vi "Private AdsSymbolVersionChanged Event Callback.vi"(4 "TwinCAT ADS out":refnum<class "TwinCAT ADS.lvclass">, 5 "Event Data":cluster{"sender":refnum<k24>, "e":refnum<k24>}, 6 "Control Ref":refnum<k24>, 7 "Event Common Data":T1) -> ()   [LabVIEW 2018, in "TwinCAT ADS.lvclass"]
uses:
  TwinCAT ADS.lvclass
  TwinCAT.Ads
  TwinCAT ADS.lvclass/TwinCAT ADS.ctl
  <vilib>/event_ctls.llb/usereventprio.ctl
  Get Type Map.vi
  From Notification Key.vi
  Get Notification Map.vi
  Extensions/Delete Notification By Handle.vi
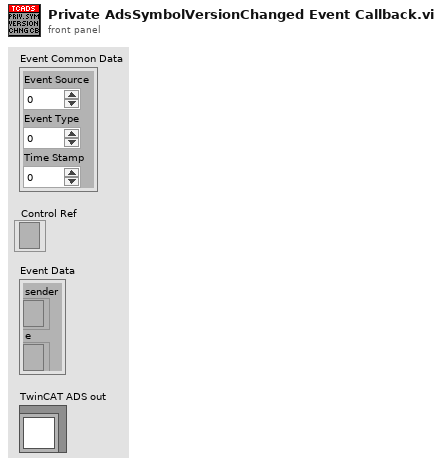
[diagram p1: front panel]
types:
  T1 = cluster{"Event Source":i32, "Event Type":u32, "Time Stamp":u32}
  T2 = typedef "usereventprio.ctl" = enum32{"high priority", "normal priority"}
  T3 = typedef "TwinCAT ADS.lvclass/Notifcation Map Value.ctl" = cluster{"Handle":i32, "Cycle Time":i32}
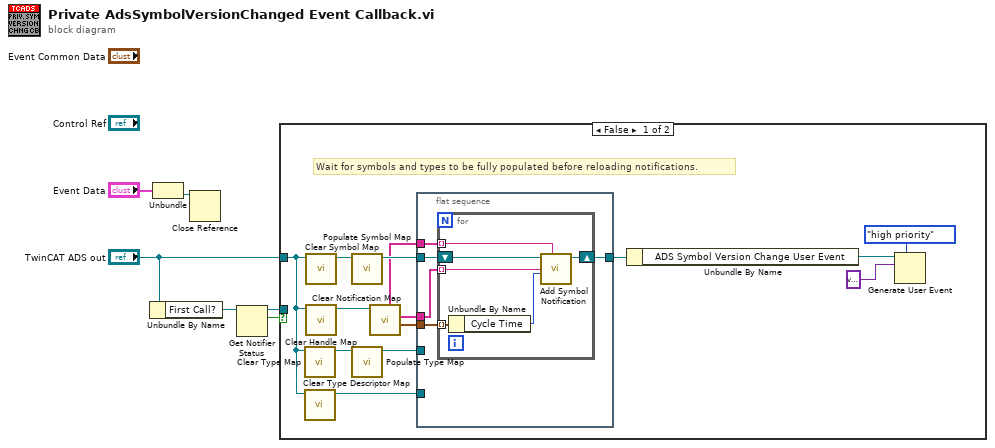
[diagram p0: block diagram]
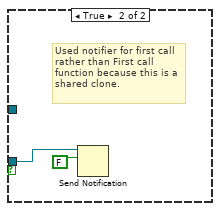
[diagram p2: hidden frame]
diagram:
  n1 = Unbundle By Name("TwinCAT ADS out") -> ("First Call?"=w3:refnum<notifier>)
  n2 = Unbundle("Event Data") -> ("e"=w5:refnum<k24>)  [unwired: 1 out]
  n3 = Close Reference(reference=w5) -> ()  [unwired: 1 in, 1 out]
  n4 = Get Notifier Status(notifier=w3) -> (notifier out=w1:refnum<notifier>, current notification=w2:bool)  [unwired: 1 in, 3 out]
  n5 = case shown="False" w2 {
    tunnel: "TwinCAT ADS out" -> [w8 _]
    tunnel: w1 -> [_ w33]
    frame False {
      # "Wait for symbols and types to be fully populated before reloading notifications."
      n6 = call "Clear Type Map.vi"("TwinCAT ADS in"=w8) -> ("TwinCAT ADS out"=w19:refnum<class "TwinCAT ADS.lvclass">)  [unwired: 8 in, 2 out]
      n7 = call "Clear Type Descriptor Map.vi"("TwinCAT ADS in"=w8) -> ("TwinCAT ADS out"=w7:refnum<class "TwinCAT ADS.lvclass">)  [unwired: 8 in, 2 out]
      n8 = call "Clear Symbol Map.vi"("TwinCAT ADS in"=w8) -> ("TwinCAT ADS out"=w20:refnum<class "TwinCAT ADS.lvclass">)  [unwired: 9 in, 1 out]
      n9 = call "Clear Handle Map.vi"("TwinCAT ADS in"=w8) -> ("TwinCAT ADS out"=w14:refnum<class "TwinCAT ADS.lvclass">)  [unwired: 9 in, 1 out]
      n10 = call "Populate Symbol Map.vi"("TwinCAT ADS in"=w20) -> ("TwinCAT ADS out"=w15:refnum<class "TwinCAT ADS.lvclass">)  [unwired: 9 in, 1 out]
      n11 = call "Populate Type Map.vi"("TwinCAT ADS in"=w19) -> ("TwinCAT ADS out"=w11:refnum<class "TwinCAT ADS.lvclass">)  [unwired: 9 in, 1 out]
      n12 = call "Clear Notification Map.vi"("TwinCAT ADS in"=w14) -> ("[Value]"=w12:T3[], "[Symbol Name]"=w13:string[], "[Alias]"=w9:string[])  [unwired: 6 in, 2 out]
      n13 = flat-sequence {
        tunnel: w15 -> [w25]
        tunnel: w13 -> [w23]
        tunnel: w12 -> [w22]
        tunnel: w11 -> [_]
        tunnel: [w24] -> w10
        tunnel: w9 -> [w21]
        tunnel: w7 -> [_]
        frame #0 {
          n14 = for {
            shift-right: [w30] -> w24
            shift-left: w25 -> [w31]
            tunnel: w23 -> [w29] mode=indexing
            tunnel: w22 -> [w28] mode=indexing
            tunnel: w21 -> [w26] mode=indexing
            n15 = Unbundle By Name(w28) -> ("Cycle Time"=w27:i32)
            n16 = call "Add Symbol Notification.vi"("Alias"=w26, "Cycle Time (ms)"=w27, "Symbol Name"=w29, "TwinCAT ADS in"=w31) -> ("TwinCAT ADS out"=w30:refnum<class "TwinCAT ADS.lvclass">)  [unwired: 6 in, 1 out]
          }
        }
      }
      n17 = Unbundle By Name(w10) -> ("ADS Symbol Version Change User Event"=w16:refnum<user-event>)
      n18 = Generate User Event(priority (normal)=usereventprio."high priority", user event=w16, event data cluster=variant ("event data")) -> ()  [unwired: 1 in, 2 out]
    }
    frame True {
      # "Used notifier for first call rather than First call function because this is a shared clone."
      n19 = Send Notification(notification=FALSE, notifier=w33) -> ()  [unwired: 1 in, 2 out]
    }
  }
